vi "RUN ARM.vi"(8 "error in (no error)":errorcluster, 10 "input cluster":T1, 11 "MotorControlDevRef in":T2) -> (0 "error out":errorcluster)   [LabVIEW 2023]
uses:
  <vilib>/Rock Robotics/WPI/MotorControl/WPI_MotorControlDeviceRef.ctl
  <vilib>/Rock Robotics/WPI/MotorControl/WPI_MotorControlType.ctl
  <vilib>/Rock Robotics/SystemInterfaces/DIO/FPGA_DIOPWMChannel.ctl
  <vilib>/Rock Robotics/WPI/PWM/WPI_PWMDeadband.ctl
  <vilib>/Rock Robotics/SystemInterfaces/DIO/FPGA_DIOChannel.ctl
  <vilib>/Rock Robotics/WPI/ThirdParty/REV Robotics/REVLib/Typedef/Spark MAX Control Type.ctl
  <vilib>/Rock Robotics/WPI/ThirdParty/REV Robotics/REVLib/Typedef/Spark MAX Limit Direction.ctl
  Global INIT.vi
panel:
  in  "ARM\nFeed Fwd":dbl=0.1
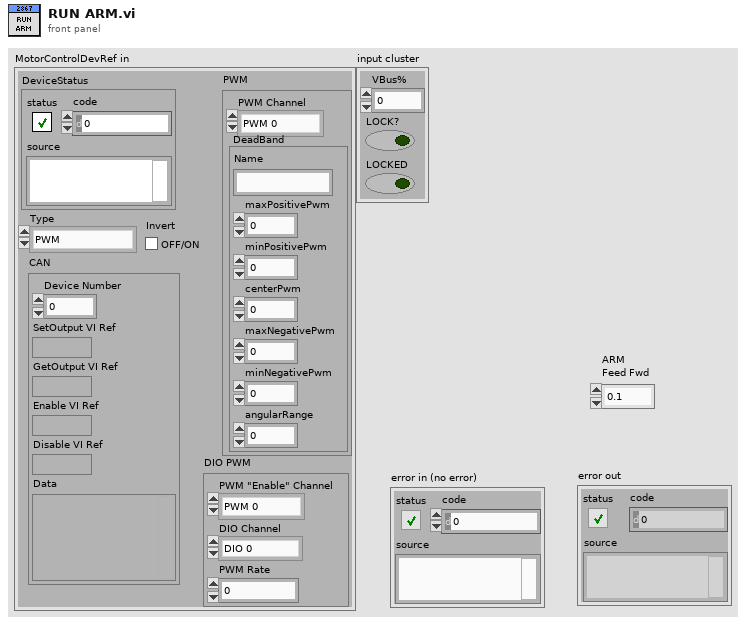
[diagram p1: front panel]
types:
  T1 = cluster{"VBus%":dbl, "LOCK?":bool, "LOCKED":bool}
  T2 = typedef "WPI_MotorControlDeviceRef.ctl" = cluster{"DeviceStatus":errorcluster, "Type":T3, "PWM":cluster{"PWM Channel":T4, "DeadBand":T5}, "CAN":cluster{"Device Number":u8, "SetOutput VI Ref":variant, "GetOutput VI Ref":variant, "Enable VI Ref":variant, "Disable VI Ref":variant, "Data":variant}, "Invert":bool, "DIO PWM":cluster{"PWM \"Enable\" Channel":T4, "DIOChannel":T6, "PWM Rate":dbl}}
  T3 = typedef "WPI_MotorControlType.ctl" = enum16{"PWM", "CAN", "DIO PWM"}
  T4 = typedef "FPGA_DIOPWMChannel.ctl" = enum8{"PWM 0", "PWM 1", "PWM 2", "PWM 3", "PWM 4", "PWM 5", "PWM 6", "PWM 7", "PWM 8", "PWM 9", "PWM MXP 0", "PWM MXP 1", "PWM MXP 2", "PWM MXP 3", "PWM MXP 4", "PWM MXP 5", "PWM MXP 6", "PWM MXP 7", "PWM MXP 8", "PWM MXP 9", "Invalid"}
  T5 = typedef "WPI_PWMDeadband.ctl" = cluster{"Name":string, "maxPositivePwm":i32, "minPositivePwm":i32, "centerPwm":i32, "maxNegativePwm":i32, "minNegativePwm":i32, "angularRange":u16}
  T6 = typedef "FPGA_DIOChannel.ctl" = enum8{"DIO 0", "DIO 1", "DIO 2", "DIO 3", "DIO 4", "DIO 5", "DIO 6", "DIO 7", "DIO 8", "DIO 9", "DIO MXP 0", "DIO MXP 1", "DIO MXP 2", "DIO MXP 3", "DIO MXP 4", "DIO MXP 5", "DIO MXP 6", "DIO MXP 7", "DIO MXP 8", "DIO MXP 9", "DIO MXP 10", "DIO MXP 11", "DIO MXP 12", "DIO MXP 13", "DIO MXP 14", "DIO MXP 15", "SPI Port CS1", "SPI Port CS2", "SPI Port CS3", "SPI Port MISO", "SPI Port MOSI", "Invalid"}
  T7 = typedef "Spark MAX Control Type.ctl" = enum16{"Percent VBus", "Voltage", "Velocity", "Position", "Smart Motion", "Current", "Smart Velocity"}
  T8 = typedef "Spark MAX Limit Direction.ctl" = enum16{"Forward Limit", "Reverse Limit"}
  T9 = typedef "ctrl intake speeds.ctl" = cluster{"forward":dbl, "reverse":dbl}
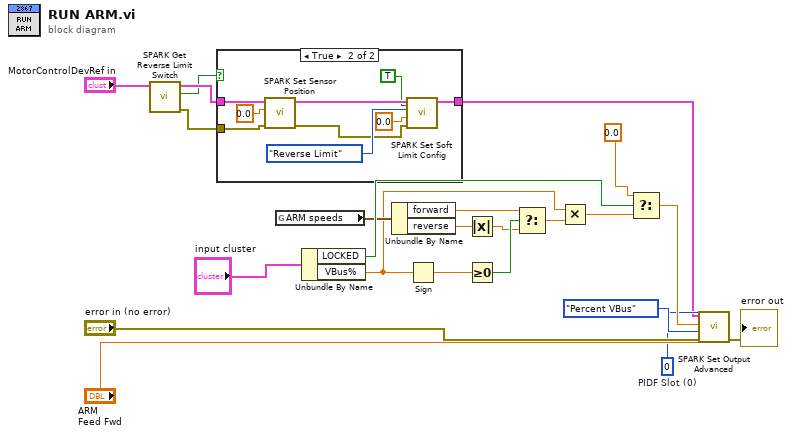
[diagram p0: block diagram]
diagram:
  w5 = 0  # PIDF Slot (0)
  n1 = call <vilib>:"SPARK Get Reverse Limit Switch.vi"("MotorControlDevRef in"="MotorControlDevRef in") -> ("error out"=w1:errorcluster, "Hard Limit Rev"=w2:bool, "MotorControlDevRef out"=w4:T2)  [unwired: 7 in, 1 out]
  n2 = case shown="True" w2 {
    tunnel: w4 -> [w24 w33]
    tunnel: [w24 w30] -> w3
    tunnel: w1 -> [_ w25]
    frame False {
    }
    frame True {
      n3 = call <vilib>:"SPARK Set Sensor Position.vi"("error in"=w25, "Position"=0.0, "MotorControlDeviceRef"=w33) -> ("error out"=w26:errorcluster, "MotorControlDeviceRef"=w31:T2)  [unwired: 7 in]
      n4 = call <vilib>:"SPARK Set Soft Limit Config.vi"("Enabled? (T)"=TRUE, "error in (no error)"=w26, "Soft Limit (0)"=0.0, "Soft Limit Switch"=Spark_MAX_Limit_Direction."Reverse Limit", "MotorControlDeviceRef in"=w31) -> ("MotorControlDeviceRef out"=w30:T2)  [unwired: 5 in, 1 out]
    }
  }
  n5 = global read "Global INIT.vi" "ARM speeds"() -> (w14:T9)
  n6 = Unbundle By Name("input cluster") -> ("LOCKED"=w18:bool, "VBus%"=w13:dbl)
  n7 = Unbundle By Name(w14) -> ("forward"=w10:dbl, "reverse"=w9:dbl)
  n8 = Sign(1:w13) -> (0:w12:dbl)
  n9 = Absolute Value(x=w9) -> (abs(x)=w7:dbl)
  n10 = Greater Or Equal To 0?(x=w12) -> (x >= 0?=w11:bool)
  n11 = Select(t=w10, s=w11, f=w7) -> (s? t:f=w8:dbl)
  n12 = Multiply(x=w13, y=w8) -> (x*y=w15:dbl)
  n13 = Select(t=0.0, s=w18, f=w15) -> (s? t:f=w19:dbl)
  n14 = call <vilib>:"SPARK Set Output Advanced.vi"("Arbitrary Feed Forward (0)"="ARM\nFeed Fwd", "PIDF Slot (0)"=w5, "error in (no error)"="error in (no error)", "Control Mode"=Spark_MAX_Control_Type."Percent VBus", "Setpoint"=w19, "MotorControlDevRef"=w3) -> ("error out"=→"error out":errorcluster)  [unwired: 4 in, 1 out]
